vi "Execute.vi"(8 "error in (no error)":errorcluster, 9 "System in":refnum<class "System.lvclass">, 10 "Command in":refnum<class "Command.lvclass">, 11 "GW-Stopping-State in":refnum<class "GW-Stopping-State.lvclass">) -> (0 "error out":errorcluster, 2 "Next State":refnum<class "State.lvclass">, 3 "GW-Stopping-State out":refnum<class "GW-Stopping-State.lvclass">)   [LabVIEW 2013, in "GW-Stopping-State.lvclass"]
uses:
  GW-Stopping-State.lvclass
  Commands/Command/Command.lvclass
  Systems/System/System.lvclass
  State/State.lvclass
  Systems/GrabberWheels/GrabberWheels.lvclass
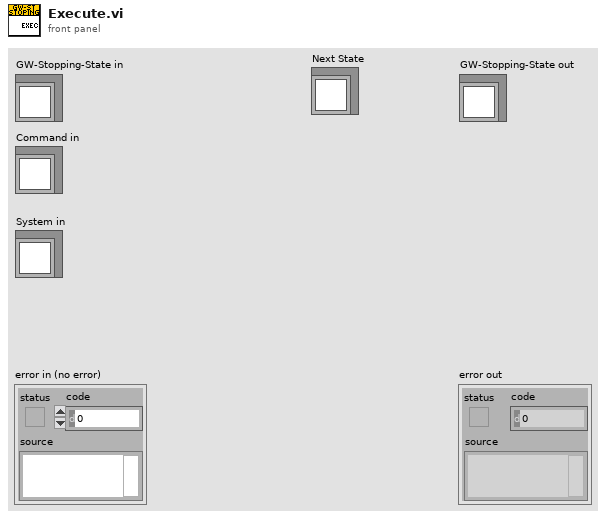
[diagram p1: front panel]
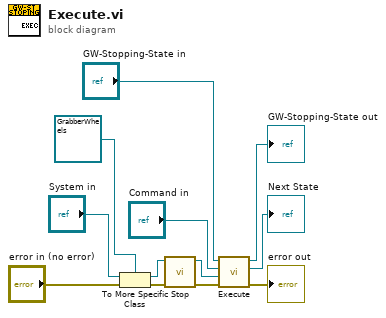
[diagram p0: block diagram]
diagram:
  n1 = To More Specific Class(target class=refnum<class "GrabberWheels.lvclass"> refnum ("GrabberWheels.lvclass"), reference="System in", error in="error in (no error)") -> (specific class reference=w4:refnum<class "GrabberWheels.lvclass">, error out=w3:errorcluster)
  n2 = call-dynamic "Stop.vi"("error in (no error)"=w3, "GrabberWheels in"=w4) -> ("error out"=w2:errorcluster, "GrabberWheels out"=w1:refnum<class "GrabberWheels.lvclass">)  [unwired: 8 in]
  n3 = call-parent "Execute.vi"("error in (no error)"=w2, "System in"=w1, "Command in"="Command in", "State in"="GW-Stopping-State in") -> ("error out"=→"error out":errorcluster, "Next State"=→"Next State":refnum<class "State.lvclass">, "State out"=→"GW-Stopping-State out":refnum<class "GW-Stopping-State.lvclass">)  [unwired: 5 in]
